vi "Datei im Ordner des VI (EXE).vi"(11 "Dateiname":string="abc") -> (0 "EXE":bool, 2 "Ordner des Haupt-VIs":path, 3 "Dateipfad im Ordner des Haupt-VIs":path)   [LabVIEW 2020, in "allgemeine Sub-VIs.lvlib"]
doc: "Erzeugt einen vollständigen Dateipfad mit dem Namens-Teil \"Dateiname\" und dem Ordner des aktuellen Hauptprogrammes, wenn das Hauptprogramm als Anwendung (.exe) läuft. Für die Entwicklungsphase muss das VI im selben Ordner wie das Haupt-VI liegen."
uses:
  Allgemein/allgemeine Sub-VIs.lvlib
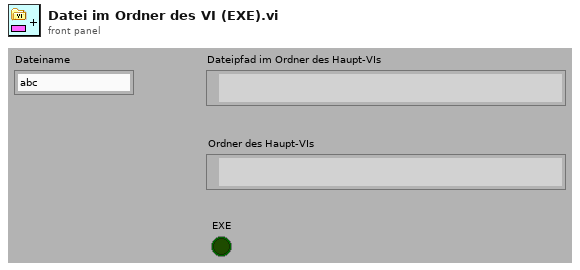
[diagram p1: front panel]
types:
  T1 = enum32{"invalid app kind", "Development System", "Run Time System", "Student Edition", "Embedded LabVIEW", "Evaluation", "Custom"}
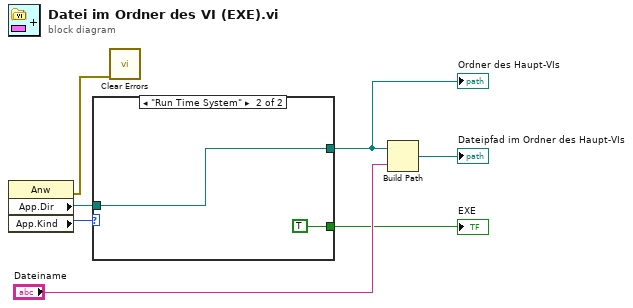
[diagram p0: block diagram]
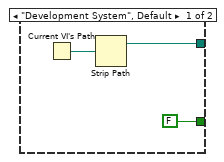
[diagram p2: hidden frame]
diagram:
  n1 = property class="Anw"() -> (error out=w1:errorcluster, "App.Dir"=w4:path, "App.Kind"=w5:T1)  [unwired: 2 in, 1 out]
  n2 = case shown="\"Run Time System\"" w5 {
    tunnel: w4 -> [_ w12]
    tunnel: [w10 w12] -> w3
    tunnel: [FALSE TRUE] -> w2
    frame "Development System", Default {
      n3 = Current VI's Path() -> (path=w8:path)
      n4 = Strip Path(path=w8) -> (stripped path=w10:path)  [unwired: 1 out]
    }
    frame "Run Time System" {
    }
  }
  "Ordner des Haupt-VIs" <- w3
  "EXE" <- w2
  n5 = call <vilib>:"Clear Errors.vi"("error in (no error)"=w1) -> ()  [unwired: 5 in, 2 out]
  n6 = Build Path(base path=w3, name or relative path="Dateiname") -> (appended path=→"Dateipfad im Ordner des Haupt-VIs":path)
